vi "FuseTargetingInformation.vi"(4 "Robot_H (deg)":dbl, 6 "LimeLight Valid":bool, 8 "LimeLight Raw Horizontal Offset (deg)":dbl, 10 "Estimated Heading to Target (deg)":dbl, 11 "Estimated Distance to Target (in)":dbl) -> (1 "Pointed at Target":bool, 2 "Fused Heading to Target Delta (deg)":dbl, 3 "Fused Distance to Target (in)":dbl)   [LabVIEW 2019]
uses:
  dsdata.vi
panel:
  in  "Min Timed Aligned (ms)":u32=200
  in  "Acceptable Heading Error (deg)":dbl=5.0
  in  "loop cycles to average":i32=15
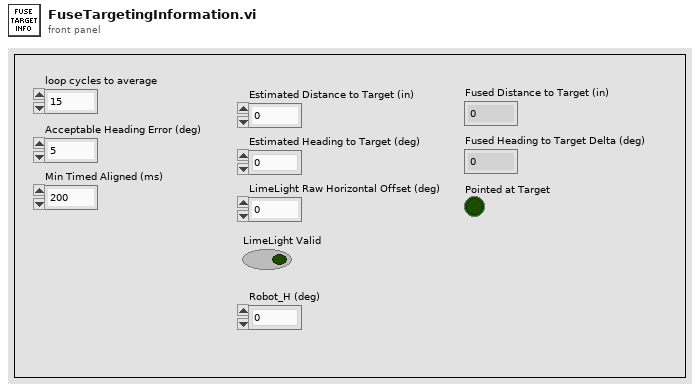
[diagram p1: front panel]
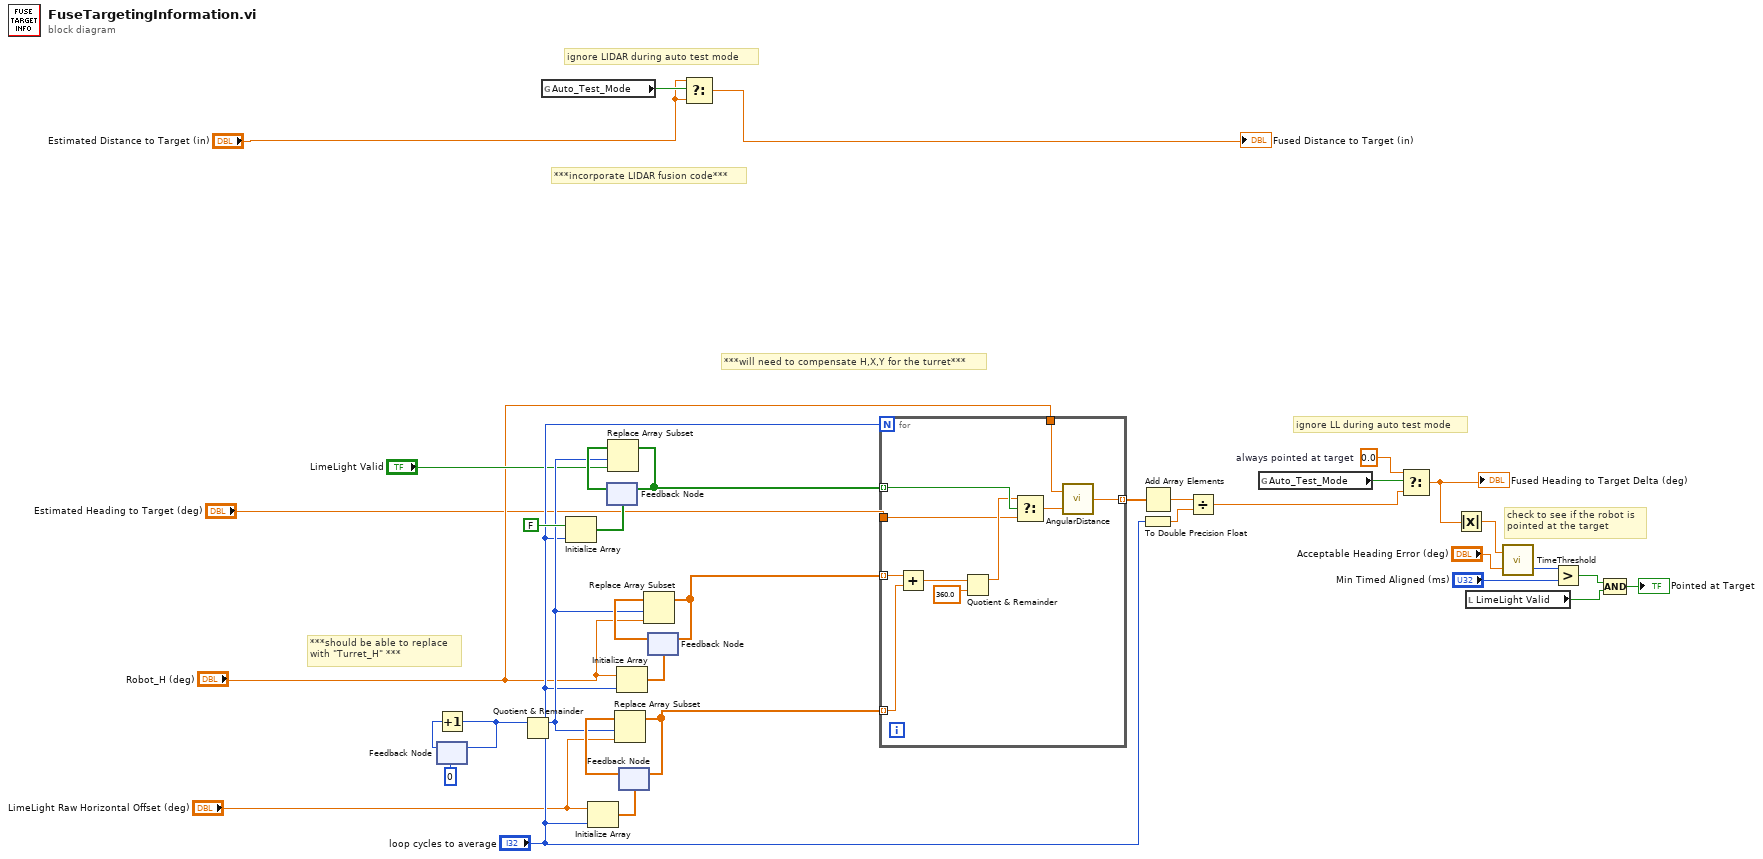
[diagram p0: block diagram]
diagram:
  w14 = 0.0  # always pointed at target
  # "check to see if the robot is\npointed at the target"
  # "***incorporate LIDAR fusion code***"
  # "ignore LIDAR during auto test mode"
  # "ignore LL during auto test mode"
  # "***should be able to replace \nwith \"Turret_H\" ***"
  # "***will need to compensate H,X,Y for the turret***"
  n1 = feedback #1(0) -> (w33:i32)
  n2 = Increment(x=w33) -> (x+1=w32:i32)
  n3 = feedback-in #1(w32) -> ()
  n4 = Quotient & Remainder(x=w32, y="loop cycles to average") -> (x-y*floor(x/y)=w24:i32)  [unwired: 1 out]
  n5 = global read "dsdata.vi" "Auto_Test_Mode"() -> (w11:bool)
  n6 = Initialize Array(FALSE, "loop cycles to average") -> (w29:bool[])
  n7 = Initialize Array("LimeLight Raw Horizontal Offset (deg)", "loop cycles to average") -> (w36:dbl[])
  n8 = feedback #2(w29) -> (w31:bool[])
  n9 = Replace Array Subset(array=w31, new element="LimeLight Valid", index=w24) -> (w28:bool[])
  n10 = feedback-in #2(w28) -> ()
  n11 = Initialize Array("Robot_H (deg)", "loop cycles to average") -> (w26:dbl[])
  n12 = feedback #3(w36) -> (w35:dbl[])
  n13 = Replace Array Subset(array=w35, new element="LimeLight Raw Horizontal Offset (deg)", index=w24) -> (w27:dbl[])
  n14 = feedback-in #3(w27) -> ()
  n15 = feedback #4(w26) -> (w25:dbl[])
  n16 = Replace Array Subset(array=w25, new element="Robot_H (deg)", index=w24) -> (w23:dbl[])
  n17 = feedback-in #4(w23) -> ()
  n18 = Select(t="Estimated Distance to Target (in)", s=w11, f="Estimated Distance to Target (in)") -> (s? t:f=→"Fused Distance to Target (in)":dbl)
  n19 = for {
    N: "loop cycles to average" -> [_]
    tunnel: w28 -> [w46] mode=indexing
    tunnel: w27 -> [w43] mode=indexing
    tunnel: "Estimated Heading to Target (deg)" -> [w41]
    tunnel: w23 -> [w40] mode=indexing
    tunnel: "Robot_H (deg)" -> [w39]
    tunnel: [w37] -> w22 mode=indexing
    n20 = Add(x=w40, y=w43) -> (x+y=w45:dbl)
    n21 = Quotient & Remainder(x=w45, y=360.0) -> (x-y*floor(x/y)=w42:dbl)  [unwired: 1 out]
    n22 = Select(t=w42, s=w46, f=w41) -> (s? t:f=w38:dbl)
    n23 = call "AngularDistance.vi"("Goal Angle (deg) [0,360]"=w38, "Current Angle (deg) [-Inf,+Inf]"=w39) -> ("Signed Angular Distance (deg) [-180,+180]"=w37:dbl)
  }
  n24 = Add Array Elements(numeric array=w22) -> (sum=w21:dbl)
  n25 = To Double Precision Float(number="loop cycles to average") -> (double precision float=w20:dbl)
  n26 = Divide(x=w21, y=w20) -> (x/y=w12:dbl)
  n27 = global read "dsdata.vi" "Auto_Test_Mode"() -> (w13:bool)
  n28 = Select(t=w14, s=w13, f=w12) -> (s? t:f=w8:dbl)
  "Fused Heading to Target Delta (deg)" <- w8
  n29 = Absolute Value(x=w8) -> (abs(x)=w7:dbl)
  n30 = local read "LimeLight Valid"() -> (w2:bool)
  n31 = call "TimeThreshold.vi"("Threshold"="Acceptable Heading Error (deg)", "Current Value"=w7) -> ("Time Below Threshold (ms)"=w5:u32)  [unwired: 1 out]
  n32 = Greater?(x=w5, y="Min Timed Aligned (ms)") -> (0:w3:bool)
  n33 = Compound Arithmetic op=AND(w3, w2) -> (→"Pointed at Target":bool)
